vi "Configure Network IP Address.vi"(8 "error in (no error)":errorcluster, 10 "IP Address (\"\")":string, 11 "VISA resource name":refnum<visa-resource-name>) -> (0 "error out":errorcluster, 3 "VISA resource name out":refnum<visa-resource-name>)   [LabVIEW 2020, in "Rohde&Schwarz CMXP Base.lvlib"]
doc: "Manually assigns one or more IPv4 addresses to the network adapter. A query returns the currently assigned addresses, irrespective of whether they have been assigned manually or via DHCP.\n\nAttribute:\nRSCMXPBASE_ATTR_CONFIGURE_NETWORK_IP_ADDRESS\n\nRemote-control command:\nSYSTem:COMMunicate:NET:IPADdress"
uses:
  <instrlib>/Rohde&Schwarz CMXP Base/Rohde&Schwarz CMXP Base.lvlib
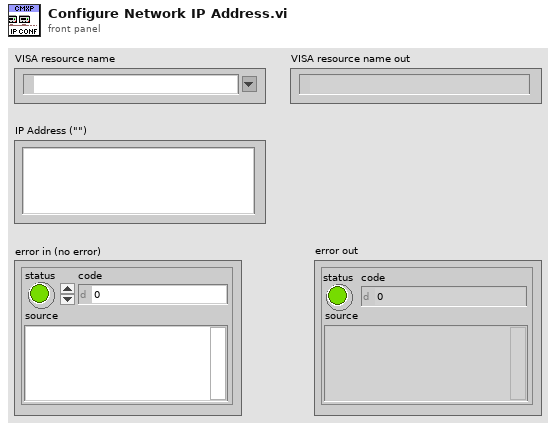
[diagram p1: front panel]
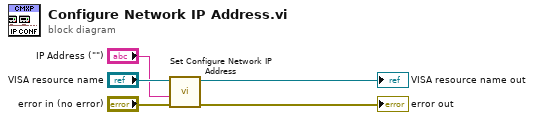
[diagram p0: block diagram]
diagram:
  n1 = call "Set Configure Network IP Address"("error in (no error)"="error in (no error)", "Configure Network IP Address ()"="IP Address (\"\")", "instrument handle"="VISA resource name") -> ("error out"=→"error out":errorcluster, "instrument handle out"=→"VISA resource name out":refnum<visa-resource-name>)  [unwired: 7 in]
